vi "Set Default Mass.vi"(8 "error in (no error)":errorcluster, 10 "Mass In":refnum<k20>, 11 "ODESimulator_LinearConveyor in":refnum<class "ODESimulator_LinearConveyor.lvclass">) -> (0 "error out":errorcluster, 2 "Mass Out":refnum<k20>, 3 "ODESimulator_LinearConveyor out":refnum<class "ODESimulator_LinearConveyor.lvclass">)   [LabVIEW 2017, in "NI_Robotics_Simulator.lvlib" / "ODESimulator_LinearConveyor.lvclass"]
uses:
  <vilib>/robotics/Simulator/Robot Factory/Conveyor/Linear/ODESimulator_LinearConveyor.lvclass
  <vilib>/robotics/Simulator/Robot Factory/Conveyor/Linear/ODESimulator_LinearConveyor.lvclass/ODESimulator_LinearConveyor.ctl
  <resource>/objmgr/LVODE.rc
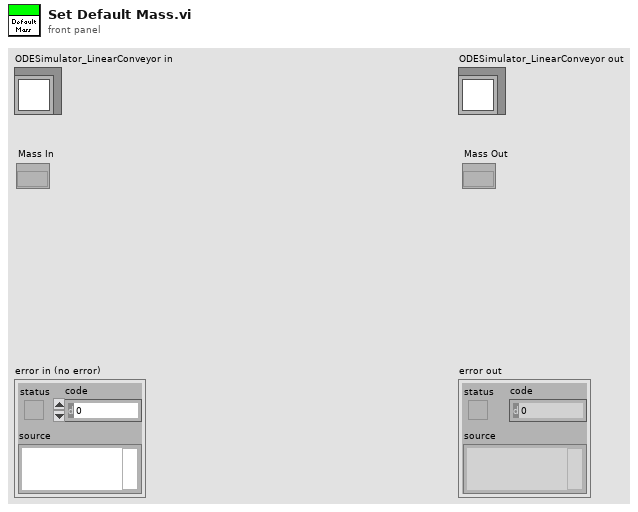
[diagram p1: front panel]
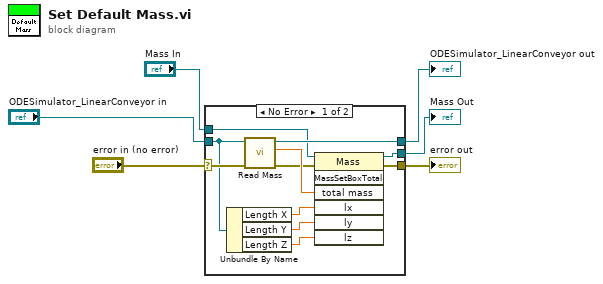
[diagram p0: block diagram]
diagram:
  n1 = case shown="No Error" "error in (no error)" {
    selector: "error in (no error)" -> [w13 w20]
    tunnel: [w8 w20] -> w1
    tunnel: [w11 w18] -> w3
    tunnel: "Mass In" -> [w10 w19]
    tunnel: [w9 w19] -> w2
    tunnel: "ODESimulator_LinearConveyor in" -> [w7 w18]
    frame No Error {
      n2 = Unbundle By Name(w7) -> ("Length X"=w17:sgl, "Length Y"=w16:sgl, "Length Z"=w15:sgl)
      n3 = call-dynamic "Read Mass.vi"("error in (no error)"=w13, "Base in"=w7) -> ("error out"=w12:errorcluster, "Mass"=w14:sgl, "Base out"=w11:refnum<class "ODESimulator_LinearConveyor.lvclass">)  [unwired: 7 in]
      n4 = invoke class="Mass" method="MassSetBoxTotal"(reference=w10, error in=w12, "total mass"=w14, "lx"=w17, "ly"=w16, "lz"=w15) -> (reference out=w9:refnum<k20>, error out=w8:errorcluster)  [unwired: 1 in, 5 out]
    }
    frame Error {
    }
  }
  "error out" <- w1
  "ODESimulator_LinearConveyor out" <- w3
  "Mass Out" <- w2
